vi "CS-4 Operate.vi"(1 "Interface (gpib)":enum16{"GPIB", "Serial"}(ring), 2 "Address":u16=1 min=1 max=31) -> (14 "dup VISA session":refnum<visa-resource-name>, 19 "error out":errorcluster)   [LabVIEW 2016]
doc: "CS-4 Operate.vi uses the CS-4 driver VI's to provide a fully functional remote interface for interactively controlling/monitoring a CS-4, and serves as an example for using the lower level VI's. When invoked it recalls the settings and starts monitoring the CS-4 readings and operational status.\n\nControl and Monitor modes are provided. When in control the supply can be remotely controlled by changing the sweep mode, units, and setup parameters.\n\nSetup parameters are changed by selecting the Setup button, and changing the sweep limits, voltage limits, sweep ranges, or sweep rates.\n\nThe remote interface to be used is specified on a pop-up menu when the program is invoked, which in turn opens a VISA channel to the specified device."
panel:
  in  "units status":enum16{"Amps", "Kilogauss", "Tesla"}(ring)=enum."Kilogauss"
  out "prev control":bool
  in  "control":bool
  out "sweep status":T1
  in  "Sweep Control":T1
  out "prev pshtr":bool
  out "pshtr status":bool
  in  "pshtr":bool
  out "Sweep Mode":string="PAUSED"
  out "Magnet Voltage":string=" +0.00 V                "
  out "Output Voltage":string=" +0.00 V                "
  out "Magnet Current":string=" +000.000 A                "
  out "Output Current":string=" +000.000 A                "
  out "Off Line":bool
  out "Power Loss":bool
  out "Quench Detect":bool
  in  "Units":enum16{"Amps", "Kilogauss", "Tesla"}(ring)
  out "Voltage Limit":dbl=5.0 min=0.0 max=10.0 format="%.2f"
  out "Upper Sweep Limit":dbl=10.0 min=-300.0 max=300.0 format="%.3f"
  out "Lower Sweep Limit":dbl=-10.0 min=-300.0 max=300.0 format="%.3f"
  out "Next Action":T2(ring)
  in  "Exit Flag":bool
  in  "stop":bool
  in  "Action":T2(ring)=enum."Recall Setup"
  in  "Monitor":bool
  in  "Setup":bool
  in  "Recall":bool
  out "Cryo Logo":bool
  # "CRYOMAGNETICS, INC."
  # "Model CS-4"
  # "Magnet Power Supply"
  # "Sweep Control"
  # "Persistent"
  # "Limits"
  # "Mode"
  # "Sweep Status"
  # "Switch Heater"
  # "Control"
  # "On"
  # "Monitor"
  # "Off"
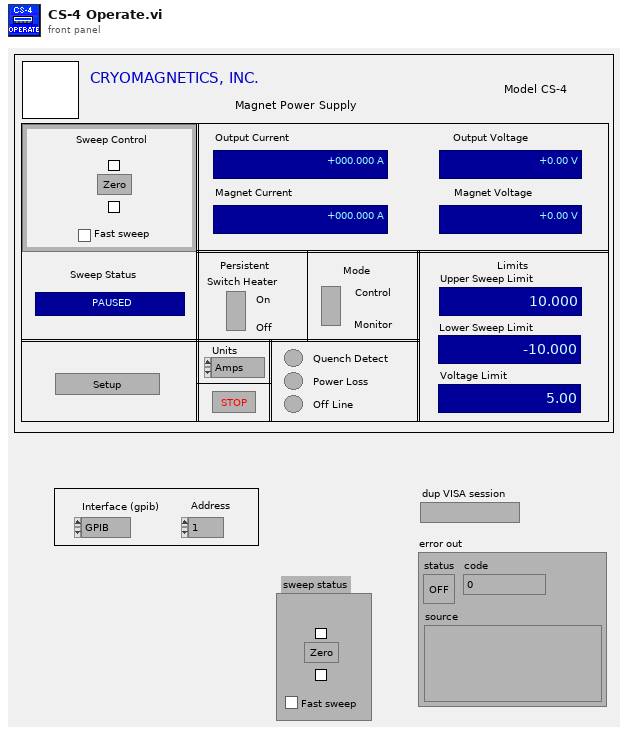
[diagram p1: front panel]
types:
  T1 = cluster{"zero":bool, "sweep up":bool, "sweep down":bool, "fast sweep":bool}
  T2 = enum16{"Idle", "Recall Setup", "Send Setup", "Monitor", "Update Limits", "Cleanup"}
  T3 = cluster{"Lower Current Limit":dbl, "Upper Current Limit":dbl, "Voltage Limit":dbl}
  T4 = cluster{"rate 0":dbl, "rate 1":dbl, "rate 2":dbl, "rate 3":dbl}
  T5 = cluster{"fast sweep":bool, "zero":bool, "sweep down":bool, "sweep up":bool}
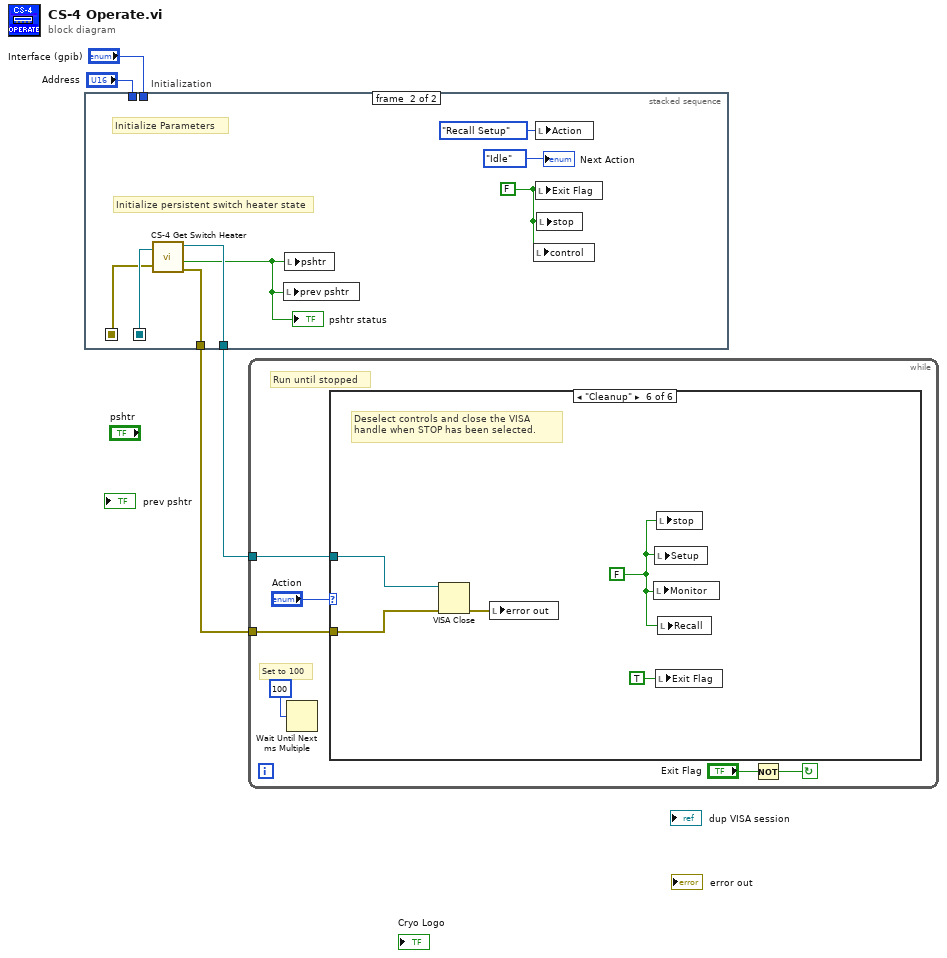
[diagram p0: block diagram]
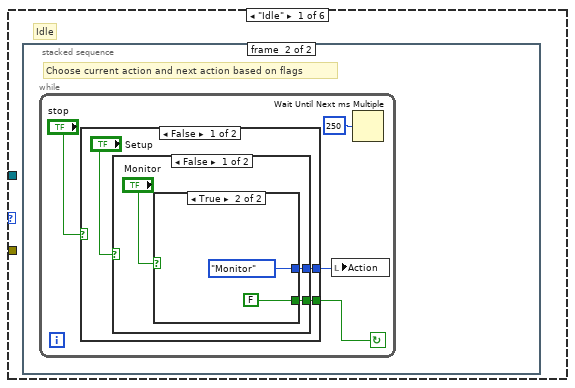
[diagram p2: hidden frame]
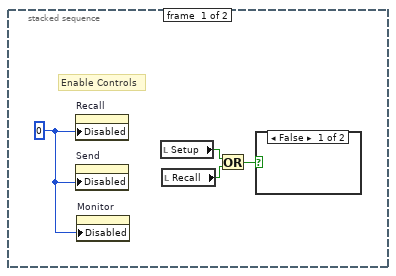
[diagram p3: hidden frame]
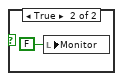
[diagram p4: hidden frame]
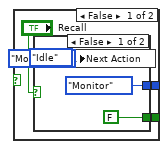
[diagram p5: hidden frame]
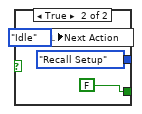
[diagram p6: hidden frame]
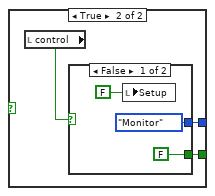
[diagram p7: hidden frame]
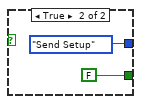
[diagram p8: hidden frame]
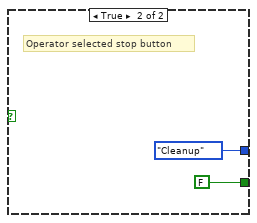
[diagram p9: hidden frame]
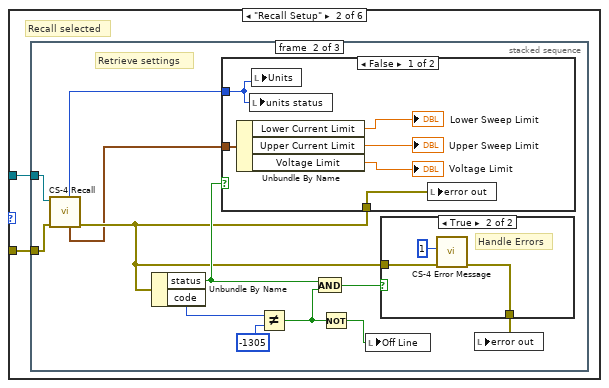
[diagram p10: hidden frame]
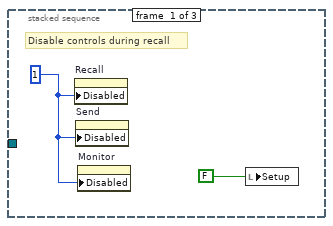
[diagram p11: hidden frame]
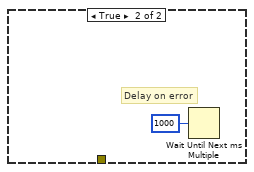
[diagram p12: hidden frame]
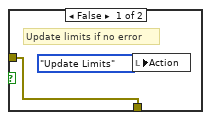
[diagram p13: hidden frame]
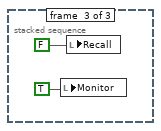
[diagram p14: hidden frame]
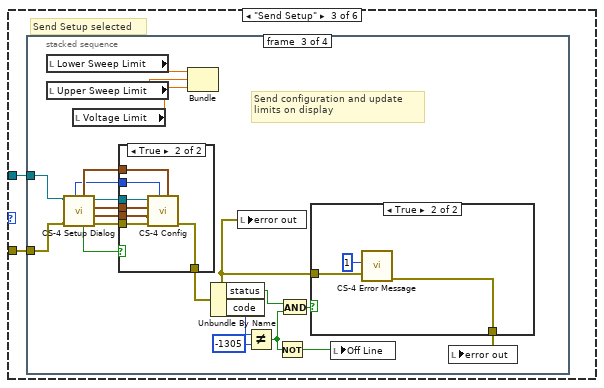
[diagram p15: hidden frame]
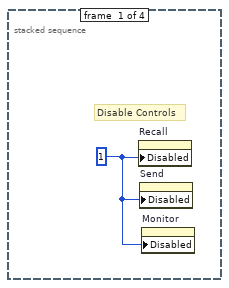
[diagram p16: hidden frame]
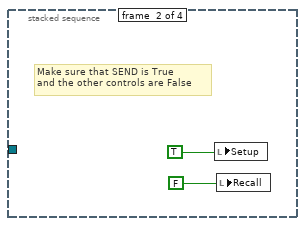
[diagram p17: hidden frame]
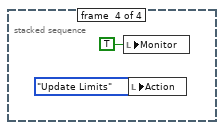
[diagram p20: hidden frame]
diagram:
  n1 = stacked-sequence "Initialization" {
    seq-local: [w6 _] -> [_ w37]
    seq-local: [w5 _] -> [_ w36]
    tunnel: [_ w35] -> w3
    tunnel: [_ w34] -> w4
    tunnel: "Address" -> [w8 _]
    tunnel: "Interface (gpib)" -> [w7 _]
    frame #0 {
      n2 = while {
        tunnel: w7 -> [w15]
        tunnel: w8 -> [w16]
        tunnel: [w10] -> w5
        tunnel: [w30] -> w6
        stop <- w14 continue-if-true
        # "2 sec delay on error"
        # "Select I/O Device"
        n3 = call "CS-4 Device.vi"("Address"=w16, "Interface"=w15) -> ("DeviceAddress"=w11:u16, "DeviceInterface"=w12:enum16{"GPIB", "Serial"})
        n4 = Equal?(x=w12, y=enum16{"GPIB", "Serial"}."Serial" ("Interface (gpib)")) -> (x = y?=w20:bool)
        n5 = local write "Address"(w11) -> ()
        n6 = Format Into String(format string="%d", initial string="ASRL", w11) -> (resulting string=w29:string)  [unwired: 1 in, 1 out]
        n7 = Format Into String(format string="%d", initial string="GPIB::", w11) -> (resulting string=w26:string)  [unwired: 1 in, 1 out]
        n8 = Select(t=w29, s=w20, f=w26) -> (s? t:f=w22:string)
        n9 = local write "Interface (gpib)"(w12) -> ()
        n10 = Concatenate Strings(w22, "::INSTR") -> (w19:string)
        n11 = call "CS-4 Initialize.vi"("Reset (T: Reset)"=FALSE ("ID Query (T: Check)"), "ID Query (T: Check)"=TRUE, "VISA session (for class)"=w19) -> ("error out"=w10:errorcluster, "VISA session"=w30:refnum<visa-resource-name>)  [unwired: 7 in]
        n12 = Unbundle By Name(w10) -> ("status"=w9:bool)
        n13 = call <vilib>:"Simple Error Handler.vi"("type of dialog (OK msg:1)"=2, "error in (no error)"=w10) -> ("error?"=w14:bool)  [unwired: 3 in, 4 out]
        n14 = case shown="True" w9 {
          frame False {
          }
          frame True {
            n15 = Wait (ms)(milliseconds to wait=u32 2000) -> ()  [unwired: 1 out]
          }
        }
      }
    }
    frame #1 {
      w32 = FALSE ("Exit Flag")
      # "Initialize persistent switch heater state"
      # "Initialize Parameters"
      n16 = call "CS-4 Get Switch Heater.vi"("VISA session"=w37, "error in (no error)"=w36) -> ("dup VISA session"=w34:refnum<visa-resource-name>, "switch heater"=w33:bool, "error out"=w35:errorcluster)  [unwired: 1 in]
      "pshtr status" <- w33
      n17 = local write "prev pshtr"(w33) -> ()
      n18 = local write "pshtr"(w33) -> ()
      n19 = local write "control"(w32) -> ()
      n20 = local write "Action"(T2."Recall Setup" ("Action")) -> ()
      n21 = local write "Exit Flag"(w32) -> ()
      n22 = local write "stop"(w32) -> ()
      "Next Action" <- T2."Idle" ("Next Action")
    }
  }
  n23 = while {
    tunnel: w4 -> [w43]
    tunnel: w3 -> [w44]
    stop <- w41 continue-if-true
    # "Set to 100"
    # "Run until stopped"
    n24 = Wait Until Next ms Multiple(millisecond multiple=u32 100) -> ()  [unwired: 1 out]
    n25 = case shown="\"Cleanup\"" "Action" {
      tunnel: w44 -> [_ w82 w113 w152 _ w339]
      tunnel: w43 -> [_ w83 w112 w151 _ w338]
      frame "Idle" {
        # "Idle"
        n26 = stacked-sequence {
          frame #0 {
            w49 = u8 0 ("Disabled")
            # "Enable Controls"
            n27 = property on="Recall" class="Bool (strict)"("Disabled"=w49) -> ()  [unwired: 2 in, 2 out]
            n28 = property on="Send" class="Bool (strict)"("Disabled"=w49) -> ()  [unwired: 2 in, 2 out]
            n29 = property on="Monitor" class="Bool (strict)"("Disabled"=w49) -> ()  [unwired: 2 in, 2 out]
            n30 = local read "Setup"() -> (w48:bool)
            n31 = local read "Recall"() -> (w47:bool)
            n32 = Or(x=w48, y=w47) -> (x .or. y?=w46:bool)
            n33 = case shown="False" w46 {
              frame False {
              }
              frame True {
                n34 = local write "Monitor"(FALSE ("Monitor")) -> ()
              }
            }
          }
          frame #1 {
            # "Choose current action and next action based on flags"
            n35 = while {
              stop <- w53 continue-if-true
              n36 = case shown="False" "stop" {
                tunnel: [w56 T2."Cleanup" ("Action")] -> w54
                tunnel: [w55 FALSE] -> w53
                frame False {
                  n37 = case shown="False" "Setup" {
                    tunnel: [w60 w74] -> w56
                    tunnel: [w59 w73] -> w55
                    frame False {
                      n38 = case shown="True" "Monitor" {
                        tunnel: [w62 T2."Monitor" ("Action")] -> w60
                        tunnel: [w61 FALSE] -> w59
                        frame False {
                          n39 = case shown="False" "Recall" {
                            tunnel: [FALSE FALSE] -> w61
                            tunnel: [T2."Monitor" ("Action") T2."Recall Setup" ("Action")] -> w62
                            frame False {
                              (unwired) T2."Monitor" ("Next Action")
                              n40 = local write "Next Action"(T2."Idle" ("Next Action")) -> ()
                            }
                            frame True {
                              n41 = local write "Next Action"(T2."Idle" ("Next Action")) -> ()
                            }
                          }
                        }
                        frame True {
                          # "If Monitor then no state change"
                        }
                      }
                    }
                    frame True {
                      n42 = local read "control"() -> (w72:bool)
                      n43 = case shown="False" w72 {
                        tunnel: [FALSE FALSE] -> w73
                        tunnel: [T2."Monitor" ("Action") T2."Send Setup" ("Action")] -> w74
                        frame False {
                          n44 = local write "Setup"(FALSE ("Setup")) -> ()
                        }
                        frame True {
                        }
                      }
                    }
                  }
                }
                frame True {
                  # "Operator selected stop button"
                }
              }
              n45 = local write "Action"(w54) -> ()
              n46 = Wait Until Next ms Multiple(millisecond multiple=u32 250) -> ()  [unwired: 1 out]
            }
          }
        }
      }
      frame "Recall Setup" {
        # "Recall selected"
        n47 = stacked-sequence {
          tunnel: w83 -> [_ w97 _]
          tunnel: w82 -> [_ w96 _]
          frame #0 {
            w85 = u8 1 ("Disabled")
            # "Disable controls during recall"
            n48 = property on="Recall" class="Bool (strict)"("Disabled"=w85) -> ()  [unwired: 2 in, 2 out]
            n49 = property on="Send" class="Bool (strict)"("Disabled"=w85) -> ()  [unwired: 2 in, 2 out]
            n50 = property on="Monitor" class="Bool (strict)"("Disabled"=w85) -> ()  [unwired: 2 in, 2 out]
            n51 = local write "Setup"(FALSE ("Send")) -> ()
          }
          frame #1 {
            # "Retrieve settings"
            n52 = call "CS-4 Recall.vi"("error in (no error)"=w96, "VISA session"=w97) -> ("error out"=w87:errorcluster, "limits"=w86:T3, "Units"=w89:enum16{"Amps", "Kilogauss", "Tesla"})  [unwired: 4 in, 3 out]
            n53 = Unbundle By Name(w87) -> ("status"=w90:bool, "code"=w88:i32)
            n54 = case shown="False" w90 {
              tunnel: w89 -> [w98 _]
              tunnel: w87 -> [w103 _]
              tunnel: w86 -> [w102 _]
              frame False {
                n55 = Unbundle By Name(w102) -> ("Lower Current Limit"=→"Lower Sweep Limit":dbl, "Upper Current Limit"=→"Upper Sweep Limit":dbl, "Voltage Limit"=→"Voltage Limit":dbl)
                n56 = local write "units status"(w98) -> ()
                n57 = local write "Units"(w98) -> ()
                n58 = local write "error out"(w103) -> ()
              }
              frame True {
                # "Delay on error"
                n59 = Wait Until Next ms Multiple(millisecond multiple=u32 1000) -> ()  [unwired: 1 out]
              }
            }
            n60 = Not Equal?(x=w88, y=-1305) -> (x != y?=w94:bool)
            n61 = And(x=w90, y=w94) -> (x .and. y?=w93:bool)
            n62 = Not(x=w94) -> (.not. x?=w91:bool)
            n63 = local write "Off Line"(w91) -> ()
            n64 = case shown="True" w93 {
              tunnel: w87 -> [w105 w109]
              tunnel: [w105 w108] -> w92
              frame False {
                # "Update limits if no error"
                n65 = local write "Action"(T2."Update Limits" ("Action")) -> ()
              }
              frame True {
                # "Handle Errors"
                n66 = call "CS-4 Error Message.vi"("error in (no error)"=w109, "Type of Dialog (1: OK Msg)"=1) -> ("error out"=w108:errorcluster)  [unwired: 5 in, 4 out]
              }
            }
            n67 = local write "error out"(w92) -> ()
          }
          frame #2 {
            n68 = local write "Monitor"(TRUE ("Send")) -> ()
            n69 = local write "Recall"(FALSE ("Send")) -> ()
          }
        }
      }
      frame "Send Setup" {
        # "Send Setup selected"
        n70 = stacked-sequence {
          tunnel: w113 -> [_ _ w126 _]
          tunnel: w112 -> [_ _ w125 _]
          frame #0 {
            w114 = u8 1 ("Disabled")
            # "Disable Controls"
            n71 = property on="Recall" class="Bool (strict)"("Disabled"=w114) -> ()  [unwired: 2 in, 2 out]
            n72 = property on="Send" class="Bool (strict)"("Disabled"=w114) -> ()  [unwired: 2 in, 2 out]
            n73 = property on="Monitor" class="Bool (strict)"("Disabled"=w114) -> ()  [unwired: 2 in, 2 out]
          }
          frame #1 {
            # "Make sure that SEND is True\nand the other controls are False"
            n74 = local write "Setup"(TRUE ("Recall")) -> ()
            n75 = local write "Recall"(FALSE ("Send")) -> ()
          }
          frame #2 {
            # "Send configuration and update\nlimits on display"
            n76 = local read "Lower Sweep Limit"() -> (w129:dbl)
            n77 = local read "Upper Sweep Limit"() -> (w128:dbl)
            n78 = call "CS-4 Setup Dialog.vi"("error in"=w126, "VISA session"=w125) -> ("error out"=w122:errorcluster, "sweep rates out"=w120:T4, "sweep range"=w121:cluster{"range 0":dbl, "range 1":dbl}, "dup VISA session"=w123:refnum<visa-resource-name>, "send"=w119:bool, "limits out"=w124:T3, "Units"=w118:enum16{"Amps", "Kilogauss", "Tesla"})  [unwired: 3 in]
            n79 = local read "Voltage Limit"() -> (w127:dbl)
            n80 = case shown="True" w119 {
              tunnel: w124 -> [_ w144]
              tunnel: w123 -> [_ w143]
              tunnel: w122 -> [w137 w142]
              tunnel: w121 -> [_ w141]
              tunnel: w120 -> [_ w140]
              tunnel: w118 -> [_ w139]
              tunnel: [w137 w138] -> w117
              frame False {
              }
              frame True {
                n81 = call "CS-4 Config.vi"("limits"=w144, "Units"=w139, "error in (no error)"=w142, "sweep rates"=w140, "sweep range"=w141, "VISA session"=w143) -> ("error out"=w138:errorcluster)  [unwired: 4 in, 1 out]
              }
            }
            n82 = Bundle("Lower Sweep Limit"=w129, "Upper Sweep Limit"=w128, "Voltage Limit"=w127) -> ()  [unwired: 1 in, 1 out]
            n83 = Unbundle By Name(w117) -> ("status"=w135:bool, "code"=w131:i32)
            n84 = local write "error out"(w117) -> ()
            n85 = Not Equal?(x=w131, y=-1305) -> (x != y?=w133:bool)
            n86 = Not(x=w133) -> (.not. x?=w132:bool)
            n87 = And(x=w135, y=w133) -> (x .and. y?=w134:bool)
            n88 = case shown="True" w134 {
              tunnel: w117 -> [w145 w148]
              tunnel: [w145 w147] -> w130
              frame False {
              }
              frame True {
                n89 = call "CS-4 Error Message.vi"("error in (no error)"=w148, "Type of Dialog (1: OK Msg)"=1) -> ("error out"=w147:errorcluster)  [unwired: 5 in, 4 out]
              }
            }
            n90 = local write "Off Line"(w132) -> ()
            n91 = local write "error out"(w130) -> ()
          }
          frame #3 {
            n92 = local write "Monitor"(TRUE ("Monitor")) -> ()
            n93 = local write "Action"(T2."Update Limits" ("Action")) -> ()
          }
        }
      }
      frame "Monitor" {
        (unwired) T2."Update Limits" ("Action")
        # "Monitor Selected"
        n94 = stacked-sequence {
          seq-local: [w154 _ _ _ _] -> [_ w180 _ _ _]
          seq-local: [_ w179 _ _ _] -> [_ _ w220 _ _]
          seq-local: [_ _ w210 _ _] -> [_ _ _ w264 _]
          seq-local: [_ _ _ w265 _] -> [_ _ _ _ w295]
          tunnel: w151 -> [w171 w181 w217 w266 w297]
          tunnel: w152 -> [w170 _ _ _ _]
          frame #0 {
            n95 = call "CS-4 Get Switch Heater.vi"("VISA session"=w171, "error in (no error)"=w170) -> ("dup VISA session"=w172:refnum<visa-resource-name>, "switch heater"=w174:bool, "error out"=w173:errorcluster)  [unwired: 1 in]
            n96 = local write "pshtr status"(w174) -> ()
            n97 = call "CS-4 Status.vi"("VISA session"=w172, "error in (no error)"=w173) -> ("Magnet Current"=→"Magnet Current":string, "Magnet Voltage"=→"Magnet Voltage":string, "Output Current"=→"Output Current":string, "Output Voltage"=→"Output Voltage":string, "Sweep Mode"=→"Sweep Mode":string, "sweep states"=→"sweep status":T5, "Off Line"=→"Off Line":bool, "Power Loss"=→"Power Loss":bool, "Quench"=→"Quench Detect":bool, "error out"=w161:errorcluster)  [unwired: 2 in, 2 out]
            n98 = Unbundle By Name(w161) -> ("status"=w158:bool, "code"=w160:i32)
            n99 = Not Equal?(x=w160, y=-1305) -> (x != y?=w157:bool)
            n100 = And(x=w158, y=w157) -> (x .and. y?=w159:bool)
            n101 = case shown="False" w159 {
              tunnel: w161 -> [w175 w178]
              tunnel: [w175 w177] -> w154
              frame False {
              }
              frame True {
                n102 = call "CS-4 Error Message.vi"("error in (no error)"=w178, "Type of Dialog (1: OK Msg)"=1) -> ("error out"=w177:errorcluster)  [unwired: 5 in, 4 out]
              }
            }
            n103 = local write "Action"(T2."Idle" ("Action")) -> ()
          }
          frame #1 {
            # "Handle Switch heater"
            n104 = Unbundle By Name(w180) -> ("status"=w182:bool)
            n105 = case shown="False" w182 {
              tunnel: w181 -> [w190 _]
              tunnel: w180 -> [w189 w209]
              tunnel: [w187 w209] -> w179
              frame False {
                # "Control mode and switch heater button changed?"
                n106 = local read "pshtr"() -> (w188:bool)
                n107 = local read "prev pshtr"() -> (w186:bool)
                n108 = local read "control"() -> (w184:bool)
                n109 = Not Equal?(x=w186, y=w188) -> (x != y?=w185:bool)
                n110 = And(x=w184, y=w185) -> (x .and. y?=w183:bool)
                n111 = case shown="False" w183 {
                  tunnel: w190 -> [_ w202]
                  tunnel: w189 -> [w192 w201]
                  tunnel: w188 -> [_ w193]
                  tunnel: [w192 w194] -> w187
                  frame False {
                    n112 = local read "pshtr status"() -> (w191:bool)
                    n113 = local write "pshtr"(w191) -> ()
                  }
                  frame True {
                    n114 = Select(t="On?", s=w193, f="Off?") -> (s? t:f=w198:string)
                    n115 = Concatenate Strings("Turn Persistent Switch Heater ", w198) -> (w196:string)
                    n116 = Two Button Dialog(message=w196) -> (T button?=w195:bool)  [unwired: 2 in]
                    n117 = case shown="False" w195 {
                      tunnel: w201 -> [w204 w208]
                      tunnel: w202 -> [_ w207]
                      tunnel: [w204 w206] -> w194
                      tunnel: w193 -> [_ w205]
                      frame False {
                        n118 = local read "pshtr status"() -> (w203:bool)
                        n119 = local write "prev pshtr"(w203) -> ()
                        n120 = local write "pshtr"(w203) -> ()
                      }
                      frame True {
                        n121 = call "CS-4 Set Switch Heater.vi"("error in (no error)"=w208, "switch heater"=w205, "VISA session"=w207) -> ("error out"=w206:errorcluster)  [unwired: 3 in, 1 out]
                      }
                    }
                  }
                }
              }
              frame True {
                # "Ignore switch heater on error"
              }
            }
          }
          frame #2 {
            n122 = local read "sweep status"() -> (w213:T1)
            n123 = local read "pshtr"() -> (w211:bool)
            n124 = Unbundle By Name(w220) -> ("status"=w219:bool)
            n125 = Cluster To Array(cluster=w213) -> (array=w212:bool[])
            n126 = Cluster To Array(cluster="Sweep Control") -> (array=w215:bool[])
            n127 = local write "prev pshtr"(w211) -> ()
            n128 = Boolean Array To Number(Boolean array=w212) -> (number=w218:u32)
            n129 = Boolean Array To Number(Boolean array=w215) -> (number=w214:u32)
            n130 = case shown="False" w219 {
              tunnel: w214 -> [w227 _]
              tunnel: w218 -> [w226 _]
              tunnel: "Sweep Control" -> [w225 _]
              tunnel: w217 -> [w224 _]
              tunnel: w213 -> [w223 _]
              tunnel: w220 -> [w222 w263]
              tunnel: [w221 w263] -> w210
              frame False {
                n131 = case shown="True" "control" {
                  tunnel: w227 -> [_ w232]
                  tunnel: w226 -> [_ w231]
                  tunnel: w225 -> [_ w236]
                  tunnel: w224 -> [_ w235]
                  tunnel: w223 -> [w230 _]
                  tunnel: w222 -> [w229 w234]
                  tunnel: [w229 w233] -> w221
                  frame False {
                    # "Remote control is not selected so copy\nthe present sweep status to the buttons"
                    n132 = local write "Sweep Control"(w230) -> ()
                  }
                  frame True {
                    n133 = Not Equal?(x=w232, y=w231) -> (x != y?=w237:bool)
                    n134 = case shown="False" w237 {
                      tunnel: w236 -> [_ w244]
                      tunnel: w235 -> [_ w249]
                      tunnel: w234 -> [w238 w248]
                      tunnel: [w238 w247] -> w233
                      tunnel: w232 -> [_ w245]
                      tunnel: w231 -> [_ w246]
                      frame False {
                      }
                      frame True {
                        # "Send sweep command\nsince remote is selected"
                        n135 = Exclusive Or(1:w246, 2:w245) -> (0:w242:u32)
                        n136 = And(x=w242, y=u32 7) -> (x .and. y?=w240:u32)
                        n137 = Not Equal To 0?(x=w240) -> (x != 0?=w239:bool)
                        n138 = case shown="True" w239 {
                          tunnel: w242 -> [_ w262]
                          tunnel: [w250 w260] -> w243
                          tunnel: w244 -> [w250 w256]
                          tunnel: w245 -> [_ w251]
                          frame False {
                          }
                          frame True {
                            n139 = And(x=w251, y=w262) -> (x .and. y?=w252:u32)
                            n140 = Number To Boolean Array(number=w252) -> (Boolean array=w261:bool[])
                            n141 = Index Array(array=w261, index=0) -> (element=w257:bool)
                            n142 = Index Array(array=w261, index=1) -> (element=w258:bool)
                            n143 = Index Array(array=w261, index=2) -> (element=w259:bool)
                            n144 = Bundle By Name(cluster=w256, "zero"=w257, "sweep up"=w258, "sweep down"=w259) -> (w260:T1)
                            n145 = local write "Sweep Control"(w260) -> ()
                          }
                        }
                        n146 = call "CS-4 Set Sweep Mode.vi"("error in (no error)"=w248, "sweep mode"=w243, "VISA session"=w249) -> ("error out"=w247:errorcluster)  [unwired: 3 in, 1 out]
                      }
                    }
                  }
                }
              }
              frame True {
                # "Ignore button change on error"
              }
            }
          }
          frame #3 {
            n147 = local read "Off Line"() -> (w269:bool)
            n148 = local read "control"() -> (w268:bool)
            n149 = And(x=w269, y=w268) -> (x .and. y?=w267:bool)
            n150 = case shown="False" w267 {
              tunnel: w266 -> [w273 _]
              tunnel: w264 -> [w272 w293]
              tunnel: [w271 w293] -> w265
              frame False {
                n151 = Not Equal?(x="Units", y="units status") -> (x != y?=w274:bool)
                n152 = case shown="True" w274 {
                  tunnel: w273 -> [_ w280]
                  tunnel: w272 -> [w276 w279]
                  tunnel: [w276 w278] -> w271
                  tunnel: "Units" -> [_ w277]
                  frame False {
                  }
                  frame True {
                    n153 = stacked-sequence {
                      tunnel: w277 -> [w282 _]
                      tunnel: [w285 _] -> w278
                      tunnel: w279 -> [w284 _]
                      tunnel: w280 -> [w283 _]
                      frame #0 {
                        n154 = local read "control"() -> (w281:bool)
                        n155 = case shown="True" w281 {
                          tunnel: w282 -> [_ w290]
                          tunnel: w283 -> [_ w289]
                          tunnel: w284 -> [w286 w288]
                          tunnel: [w286 w287] -> w285
                          frame False {
                          }
                          frame True {
                            n156 = call "CS-4 Set Units.vi"("error in (no error)"=w288, "units"=w290, "VISA session"=w289) -> ("error out"=w287:errorcluster)  [unwired: 1 in, 1 out]
                          }
                        }
                      }
                      frame #1 {
                        n157 = local write "Monitor"(FALSE ("Monitor")) -> ()
                        n158 = local write "Action"(T2."Recall Setup" ("Next Action")) -> ()
                      }
                    }
                  }
                }
              }
              frame True {
                # "If instrument placed in\nlocal then go offline"
                n159 = local write "control"(FALSE ("control")) -> ()
              }
            }
          }
          frame #4 {
            n160 = local read "prev control"() -> (w299:bool)
            n161 = local read "control"() -> (w300:bool)
            n162 = Not Equal?(x=w300, y=w299) -> (x != y?=w298:bool)
            n163 = case shown="False" w298 {
              tunnel: w300 -> [_ w312]
              tunnel: w297 -> [_ w319]
              tunnel: w295 -> [w307 w318]
              tunnel: [w307 w308] -> w296
              frame False {
                # "If no change to control mode then nothing to do"
              }
              frame True {
                # "If serial interface selected\nsend local/remote on \nmode change"
                n164 = property class="Instr"(reference=w319, error in=w318) -> (reference out=w314:refnum<visa-resource-name>, error out=w313:errorcluster, "Interface Information:Interface Type"=w317:u16)
                n165 = Select(t="remote", s=w312, f="local") -> (s? t:f=w309:string)
                n166 = Equal?(x=w317, y=u16 4) -> (x = y?=w315:bool)
                n167 = case shown="True" w315 {
                  tunnel: w314 -> [_ w322]
                  tunnel: w313 -> [w320 w324]
                  tunnel: w309 -> [_ w321]
                  tunnel: [w320 w323] -> w308
                  frame False {
                  }
                  frame True {
                    n168 = call "CS-4 Write.vi"("error in (no error)"=w324, "write buffer (\"\")"=w321, "VISA session"=w322) -> ("error out"=w323:errorcluster)  [unwired: 2 out]
                  }
                }
                "prev control" <- w312
              }
            }
            n169 = Unbundle By Name(w296) -> ("status"=w304:bool, "code"=w306:i32)
            n170 = Not Equal?(x=w306, y=-1305) -> (x != y?=w303:bool)
            n171 = And(x=w304, y=w303) -> (x .and. y?=w305:bool)
            n172 = case shown="False" w305 {
              tunnel: w296 -> [w325 w328]
              tunnel: [w325 w327] -> w301
              frame False {
              }
              frame True {
                n173 = call "CS-4 Error Message.vi"("error in (no error)"=w328, "Type of Dialog (1: OK Msg)"=1) -> ("error out"=w327:errorcluster)  [unwired: 5 in, 4 out]
              }
            }
            n174 = local write "error out"(w301) -> ()
          }
        }
      }
      frame "Update Limits" {
        n175 = local read "Setup"() -> (w329:bool)
        n176 = case shown="False" w329 {
          tunnel: [w331 T2."Recall Setup" ("Next Action")] -> w330
          frame False {
            n177 = local read "Next Action"() -> (w331:T2)
          }
          frame True {
            n178 = local write "Next Action"(T2."Idle" ("Next Action")) -> ()
            n179 = local write "Setup"(FALSE ("Send")) -> ()
          }
        }
        n180 = local write "Action"(w330) -> ()
      }
      frame "Cleanup" {
        w335 = FALSE ("Exit Flag")
        # "Deselect controls and close the VISA\nhandle when STOP has been selected."
        n181 = VISA Close(VISA resource name=w338, error in (no error)=w339) -> (error out=w337:errorcluster)
        n182 = local write "error out"(w337) -> ()
        n183 = local write "Monitor"(w335) -> ()
        n184 = local write "Setup"(w335) -> ()
        n185 = local write "Exit Flag"(TRUE ("Exit Flag")) -> ()
        n186 = local write "stop"(w335) -> ()
        n187 = local write "Recall"(w335) -> ()
      }
    }
    n188 = Not(x="Exit Flag") -> (.not. x?=w41:bool)
  }
